vi "splitSchedule.vi"(10 "Schedule":T1(array[cluster])) -> (1 "Sampling Rates":dbl[](array[numeric]), 2 "Ramp Rates":T2(array[cluster]))   [LabVIEW 2018]
panel:
  # "Input: Schedule from front panel\nOutput: Ramp Rate Profile, Sampling Rate (Resolutions)"
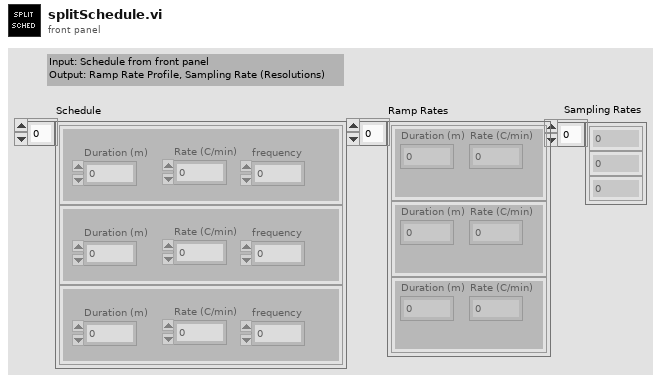
[diagram p1: front panel]
types:
  T1 = cluster{"Duration (m)":dbl, "Rate (C/min) ":dbl, "frequency":dbl}[]
  T2 = cluster{"Duration (m)":dbl, "Rate (C/min)":dbl}[]
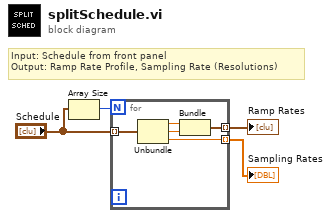
[diagram p0: block diagram]
diagram:
  # "Input: Schedule from front panel\nOutput: Ramp Rate Profile, Sampling Rate (Resolutions)"
  n1 = Array Size(array="Schedule") -> (size(s)=w4:i32)
  n2 = for {
    N: w4 -> [_]
    tunnel: "Schedule" -> [w9] mode=indexing
    tunnel: [w8] -> w1 mode=indexing
    tunnel: [w5] -> w2 mode=indexing
    n3 = Unbundle(w9) -> ("Duration (m)"=w7:dbl, "Rate (C/min)"=w6:dbl, "frequency"=w8:dbl)
    n4 = Bundle("Duration (m)"=w7, "Rate (C/min)"=w6) -> (w5:cluster{"Duration (m)":dbl, "Rate (C/min) ":dbl})  [unwired: 1 in]
  }
  "Sampling Rates" <- w1
  "Ramp Rates" <- w2
